vi "BluetothReadHost.vi"() -> ()   [LabVIEW 2010]
uses:
  <vilib>/NXT/Block Support/NXT_MessageMailbox.ctl
panel:
  out "Message":string
  in  "Stop":bool
  out "data?":bool
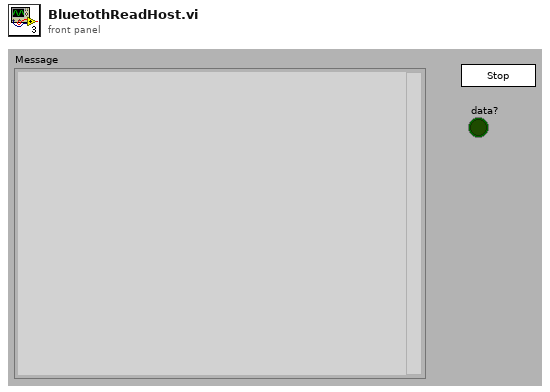
[diagram p1: front panel]
types:
  T1 = typedef "NXT_MessageMailbox.ctl" = u8
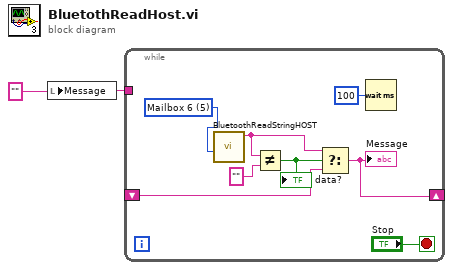
[diagram p0: block diagram]
diagram:
  w1 = "" ("Message")
  n1 = local write "Message"(w1) -> ()
  n2 = while {
    shift-right: [w2] -> _
    shift-left: _ -> [w5]
    tunnel: w1 -> [_]
    stop <- "Stop" stop-if-true
    w3 = T1 5 items=["Mailbox 1", "Mailbox 2", "Mailbox 3", "Mailbox 4", "Mailbox 5", "Mailbox 6", "Mailbox 7", "Mailbox 8", "Mailbox 9", "Mailbox 10"] ("Mailbox")
    n3 = call "BluetoothReadStringHOST.vi"("Mailbox"=w3) -> ("Message"=w4:string)  [unwired: 9 in, 1 out]
    n4 = Not Equal?(x=w4, y="") -> (x != y?=w6:bool)
    "data?" <- w6
    n5 = Select(t=w4, s=w6, f=w5) -> (s? t:f=w2:string)
    "Message" <- w2
    n6 = Wait (ms)(milliseconds to wait=u32 100) -> ()  [unwired: 1 out]
  }
